vi "Remove Enqueuer by Name.vi"(8 "error in (no error)":errorcluster, 10 "Enqueuer Name":string, 11 "Enqueuer Look Up Table in":refnum<class "Enqueuer Look Up Table.lvclass">) -> (0 "error out":errorcluster, 2 "Found?":bool, 3 "Enqueuer Look Up Table out":refnum<class "Enqueuer Look Up Table.lvclass">)   [LabVIEW 2016, in "Stream Mediator.lvlib" / "Enqueuer Look Up Table.lvclass"]
doc: "--\nCopyright © 2017 Composed SystemsI All rights reserved.\n\nAuthor: Jon McBee <jon.mcbee@composed.io>\n\nThis library is provided \"AS IS\" ,WITHOUT WARRANTIES OR\nCONDITIONS OF ANY KIND, either express or implied.\n\nComposed Systems -- composed.io\n\nStream 0.0.1.1\nJon McBee - Composed Systems\nCopyright (c) 2017, Composed Systems"
uses:
  <userlib>/Composed Systems/Stream/Mediator/Classes/Enqueuer Look Up Table/Enqueuer Look Up Table.lvclass
  C:/Program Files (x86)/National Instruments/LabVIEW 2016/user.lib/Composed Systems/Stream/Look Up Table/Look Up Table/Look Up Table.lvclass
  <userlib>/Composed Systems/Stream/Look Up Table/Look Up Table/Look Up Table.lvclass
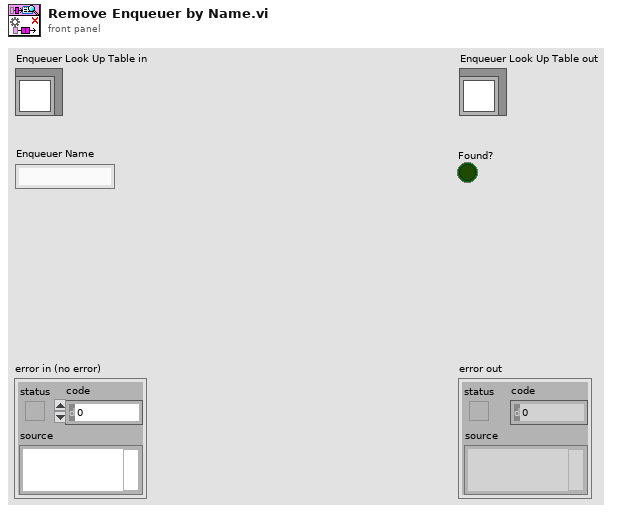
[diagram p1: front panel]
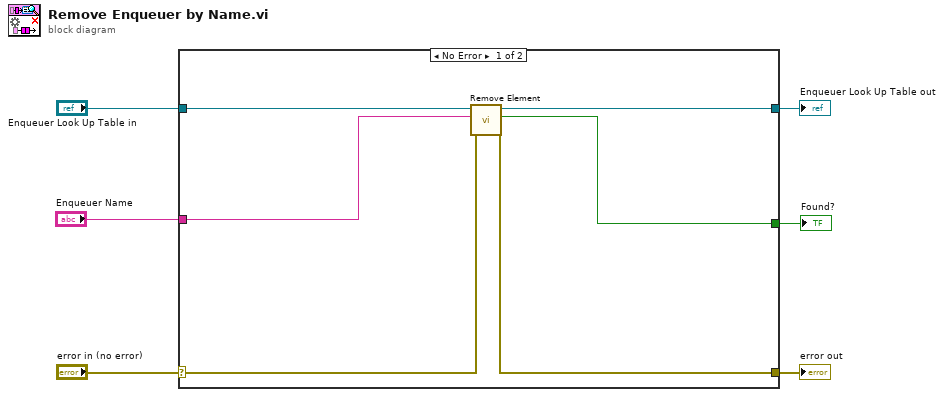
[diagram p0: block diagram]
diagram:
  n1 = case shown="No Error" "error in (no error)" {
    selector: "error in (no error)" -> [w10 w14]
    tunnel: [w9 w14] -> w5
    tunnel: [w11 w13] -> w3
    tunnel: "Enqueuer Look Up Table in" -> [w12 w13]
    tunnel: "Enqueuer Name" -> [w8 _]
    tunnel: [w7 _] -> w1
    frame No Error {
      n2 = call <userlib>:"Remove Element.vi"("error in (no error)"=w10, "Name"=w8, "Look Up Table in"=w12) -> ("error out"=w9:errorcluster, "Found?"=w7:bool, "Look Up Table out"=w11:refnum<class "Enqueuer Look Up Table.lvclass">)  [unwired: 6 in]
    }
    frame Error {
    }
  }
  "error out" <- w5
  "Enqueuer Look Up Table out" <- w3
  "Found?" <- w1
